vi "DAQmx_Settings_NI9239_v2.vi"(7 "minimum value":dbl=-5.0 format="%0.2f", 8 "error in":errorcluster, 9 "rate":dbl=1000.0 format="%0.2f", 10 "samples per channel":i32=1000, 11 "maximum value":dbl=5.0 format="%0.2f") -> (0 "error out":errorcluster, 3 "task out":refnum<k21>)   [LabVIEW 2018]
uses:
  <vilib>/DAQmx/create/channels.llb/DAQmx Create Channel (AI-Voltage-Basic).vi
  <vilib>/DAQmx/configure/timing.llb/DAQmx Timing (Sample Clock).vi
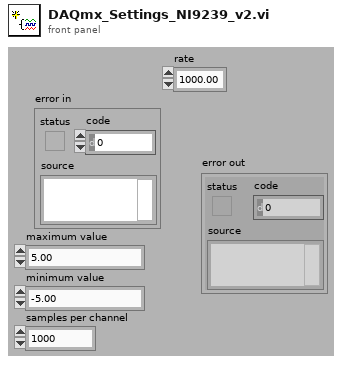
[diagram p1: front panel]
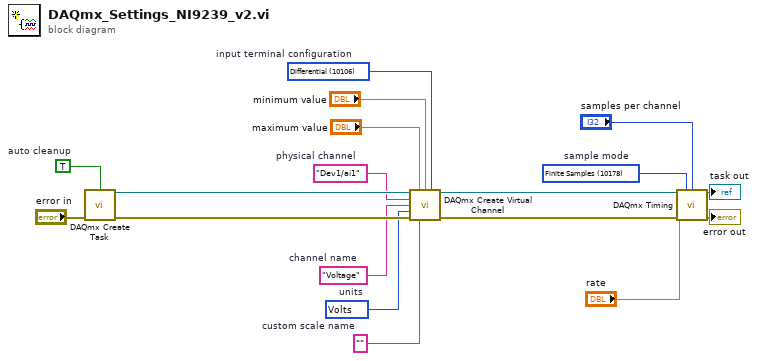
[diagram p0: block diagram]
diagram:
  w5 = 10178 items=["Finite Samples"=10178, "Continuous Samples"=10123, "Hardware Timed Single Point"=12522]  # sample mode
  w9 = 10106 items=["default"=-1, "RSE"=10083, "NRSE"=10078, "Differential"=10106, "Pseudodifferential"=12529]  # input terminal configuration
  w10 = 10348 items=["Volts"=10348, "From Custom Scale"=10065]  # units
  w11 = "Voltage"  # channel name
  w13 = ""  # custom scale name
  w14 = "Dev1/ai1"  # physical channel
  w16 = TRUE  # auto cleanup
  n1 = call <vilib>:"DAQmx Create Task.vi"("auto cleanup"=w16, "error in"="error in") -> ("task out"=w15:refnum<k21>, "error out"=w17:errorcluster)  [unwired: 12 in]
  n2 = call-poly <vilib>:"DAQmx Create Virtual Channel.vi"("task in"=w15, "maximum value"="maximum value", "minimum value"="minimum value", "input terminal configuration"=w9, "physical channels"=w14, "name to assign"=w11, "units"=w10, "error in"=w17, "custom scale name"=w13) -> ("task out"=w6:refnum<k21>, "error out"=w12:errorcluster)  [unwired: 5 in]
  n3 = call-poly <vilib>:"DAQmx Timing.vi"("task/channels in"=w6, "sample mode"=w5, "samples per channel"="samples per channel", "rate"="rate", "error in"=w12) -> ("task out"=→"task out":refnum<k21>, "error out"=→"error out":errorcluster)  [unwired: 9 in]
